vi "Micro-PL v10.2.2.vi"() -> ()   [LabVIEW 2010]
uses:
  drivers/Oxford ITC/ITCAPPS.LLB/ITCSetup.ctl
  drivers/Oxford ITC/ITCSUBS.LLB/ITCIO.ctl
  drivers/Oxford ITC/BUSGEN.LLB/OxfordAddress.ctl
  drivers/Oxford ITC/ITCSUBS.LLB/ITCVersion.ctl
  subvi/ESA-C/TypeDefs/ESA-C Live Controls.ctl
  subvi/ESA-C/TypeDefs/ESA-C Current Values.ctl
  subvi/ESA-C/TypeDefs/ESA-C Connection Settings.ctl
  subvi/ESA-C/TypeDefs/ESA-C Set Positions.ctl
  subvi/ITC503/TypeDefs/ITC503 Settings.ctl
  subvi/ITC503/TypeDefs/ITC503 Current Values.ctl
  subvi/iHR550/TypeDefs/iHR Current Values.ctl
  subvi/iHR550/TypeDefs/iHR Settings.ctl
  subvi/Mapping/TypeDefs/Mapping Spectra Params.ctl
  <vilib>/Utility/miscctls.llb/LVBoundsTypeDef.ctl
  <vilib>/Utility/miscctls.llb/LVPointTypeDef.ctl
  drivers/Horiba Spectrum One 3000V/Lib/CCD_command.llb/Comm Params.ctl
panel:
  out "Copy Drive Target":bool
  in  "CCD3500 Shutter":bool caption="Shutter:"
  out "ITC503 Temp Storage":dbl
  out "Runtime":u32
  out "ITC Gradient Time":i64
  out "Read ITC":bool
  out "Read CCD3500":bool
  out "Read iHR550":bool
  out "Read Drive":bool
  out "Spectrum Properties":cluster{"Position":T1, "Plot Area Size":T1}={"Position"={"Width"=36, "Height"=367}, "Plot Area Size"={"Width"=496, "Height"=264}}
  in  "Auto Folder":path caption="Ausgewählter Pfad"
  out "Int. Time Temp":dbl
  out "Wavelengths (nm)":dbl[](array[numeric])
  out "Measurement Running":bool
  out "ITC503s Running":bool
  out "Drive Running":bool
  out "CCD3500V Running":bool
  out "iHR550 Running":bool
  in  "Exit":bool
  out "iHR550 Status":bool
  out "Drive Status":bool
  out "CCD3500V Status":bool
  out "ITC503 Status":bool
  in  "CCD3500V Connection":T2={"Comm Interface"=1, "BUS"=0, "Address"=5, "Com Port"=0}
  out "Video Running":bool
  out "iHR550 RefNum":refnum<k7> caption="Mono RefNum out"
  out "ITC Setup":T3={"Description"="", "IO Info"={"Address"={"Com Port"=1, "ISOBUS Address"=1, "GPIB Address"=24, "Communication"=enum."ISOBUS"}, "Version"=enum."ITC503", "Ch 1 dec places"=1, "Ch 2 dec places"=1, "Ch 3 dec places"=1, "Ch1 Name"="", "Ch2 Name"="", "Ch3 Name"=""}}
  in  "Register":enum32{"Devices", "Acquisition / Mapping"}(tab)
  out "CCD3500 Temperature":dbl caption="Temp. (°C)" min=10.0 max=160.0 step=0.1 format="%.1f"
  in  "CCD3500V GPIB-Port":i32=5 caption="GPIB-Port" min=1 max=20 step=1 format="%#.0f"
  in  "CCD3500V Connect":bool
  out "CCD Timing":u32 caption="CCD"
  out "ITC Timing":u32 caption="ITC"
  out "Drive Timing":u32 caption="Drive"
  out "iHR550 Timing":u32 caption="iHR550"
  in  "iHR550 Force Init":bool=TRUE
  in  "iHR550 Connect":bool
  in  "iHR550 ID":string(combo)="iHR550" caption="Monochromator ID"
  out "ITC503 Current Values":T7 {"ITC503 Gradient" format="%.2f"; "ITC503 Setpoint" min=-273.0 max=300000.0 step=0.0001 format="%.1f"; "ITC503 I" format="%_1f"; "ITC503 P" format="%_1f"; "ITC503 Temperature" min=0.0 max=1645.0 step=1e-05 format="%.2f"; "ITC503 Heater" min=0.0 max=100.0 step=0.01 scale=0.0..100.0}
  in  "ITC503 Settings":T8={"ITC503 Set Setpoint"=0.0, "ITC503 Set Auto Heater"=TRUE, "ITC503 Set Auto PID"=TRUE, "P"=0.0, "I"=0.0, "D"=0.0} {"D" min=0.0 max=100.0 step=0.1 format="%.1f"; "I" min=0.0 max=100.0 step=0.1 format="%.1f"; "P" min=0.0 max=100.0 step=0.1 format="%.1f"; "ITC503 Set Setpoint" min=-273.0 max=300000.0 step=0.1 format="%.1f"}
  in  "ITC503 Configure":bool
  in  "ITC503 Connect":bool
  in  "ITC503 Selector":u16(ring) caption="Select Device" items=["ITC503s"]
  out "Drive Current Values":T9 {"Position"."Drive Z Position" min=-273.0 max=300000.0 step=0.0001 format="%.1f"; "Position"."Drive Y Position" min=-273.0 max=300000.0 step=0.0001 format="%.1f"; "Position"."Drive X Position" min=-273.0 max=300000.0 step=0.0001 format="%.1f"; "Voltages"."Drive Z Voltage" min=-273.0 max=300000.0 step=0.0001 format="%.1f"; "Voltages"."Drive Y Voltage" min=-273.0 max=300000.0 step=0.0001 format="%.1f"; "Voltages"."Drive X Voltage" min=-273.0 max=300000.0 step=0.0001 format="%.1f"}
  in  "Drive Connection":T10={"Objective GPIB-Port"=4, "Stage GPIB-Port"=4, "Drive Selector"=0, "Drive Velocity (V/s)"=5.0} {"Drive Velocity (V/s)" min=10.0 max=160.0 step=0.1 format="%.1f"; "Drive Selector" items=["Obj.", "Stage"]; "Stage GPIB-Port" min=1 max=20 step=1 format="%#.0f"; "Objective GPIB-Port" min=1 max=20 step=1 format="%#.0f"}
  in  "Drive Connect":bool
  in  "CCD3000 Current Rep.":string="0/0"
  in  "Spectrum Maximize":bool
  out "Spectrum":cluster{dbl[], dbl[]}[](graph)
  in  "Spectrum Load":bool
  in  "Spectrum Save":bool
  in  "Video Show":bool
  in  "Drive GoTo":bool caption="Objective Move Abs."
  in  "Drive New Positions":T11 {"Drive X Set" min=10.0 max=160.0 step=0.1 format="%.1f"; "Drive Z Set" min=10.0 max=160.0 step=0.1 format="%.1f"; "Drive Y Set" min=10.0 max=160.0 step=0.1 format="%.1f"}
  in  "Spectrum Autosave":bool caption="iHR550 Force Init"
  in  "CCD3500 Preview":bool
  in  "CCD3500 Acquire":bool
  in  "Spectra Settings":T12={"Integration Time"=1.0, "Repetitions"=1, "Mapping Spectra"=TRUE} caption="Mapping Spectra Settings" {"Repetitions" min=1 max=100 step=1; "Integration Time" min=0.1 max=6000.0 step=0.1 format="%.1f"}
  in  "Mapping Start":bool
  in  "iHR550 Configure":bool
  in  "iHR Settings":T13={"iHR550 Set Exit Mirror"=2, "iHR550 Set Side Exit"=0.0, "iHR550 Set Front Entrance"=0.0, "iHR550 Set Wavelength"=897.9988, "iHR550 Set Grating"=0, "iHR550 Set Grating Switch"=FALSE, "iHR550 Set Wavelength Switch"=FALSE, "iHR550 Set Mirror Switch"=FALSE, "iHR550 Set Slits Switch"=FALSE} {"iHR550 Set Grating" items=["1800"=1, "600"=2, "150"=3]; "iHR550 Set Wavelength" min=0.0 max=1500.0 step=1.0; "iHR550 Set Side Exit" min=0.0 max=2000.0 step=1.0; "iHR550 Set Exit Mirror" items=["Front"=2, "Side"=3]}
  out "iHR Current Values":T14={"iHR 550 Front Entrance"=0.0, "iHR550 Side Exit"=0.0, "iHR550 Wavelength"=897.9988, "iHR550 Exit Mirror"=2, "iHR550 Grating"="1", "Grating Index"=1} {"iHR550 Exit Mirror" items=["EntranceMirror", "ExitMirror", "Front", "Side"]}
  out "Drive Live Current Values":T9 {"Position"."Drive Z Position" min=-273.0 max=300000.0 step=0.0001 format="%.1f"; "Position"."Drive Y Position" min=-273.0 max=300000.0 step=0.0001 format="%.1f"; "Position"."Drive X Position" min=-273.0 max=300000.0 step=0.0001 format="%.1f"; "Voltages"."Drive Z Voltage" min=-273.0 max=300000.0 step=0.0001 format="%.1f"; "Voltages"."Drive Y Voltage" min=-273.0 max=300000.0 step=0.0001 format="%.1f"; "Voltages"."Drive X Voltage" min=-273.0 max=300000.0 step=0.0001 format="%.1f"}
  in  "Drive Live Controls":T15={"Snapshot"=FALSE, "Move Step"=1.0, "Move Home"=FALSE, "Move Down"=FALSE, "Move Up"=FALSE, "Move Left"=FALSE, "Move Right"=FALSE, "Move Out"=FALSE, "Move In"=FALSE} {"Move Step" min=0.0 max=30.0 step=0.1 format="%.1f"}
  # "Correlation Setup"
  # "Active"
  # "Active"
  # "ITC"
  # "iHR"
  # "Drive"
  # "CCD"
  # "Status"
  # "CCD"
  # "ITC"
  # "iHR"
  # "Drive"
  # "CCD"
  # "Timing"
  # "Monochromator"
  # "Cryostat"
  # "Drives"
  # "Drive Control"
  # "Spectrum"
  # "CCD"
  # "Mapping"
  # "Launch the Spectral Mapping VI and Raman Tool Set 2.0 in a new window."
  # "Monochromator"
  # "XY"
  # "Z"
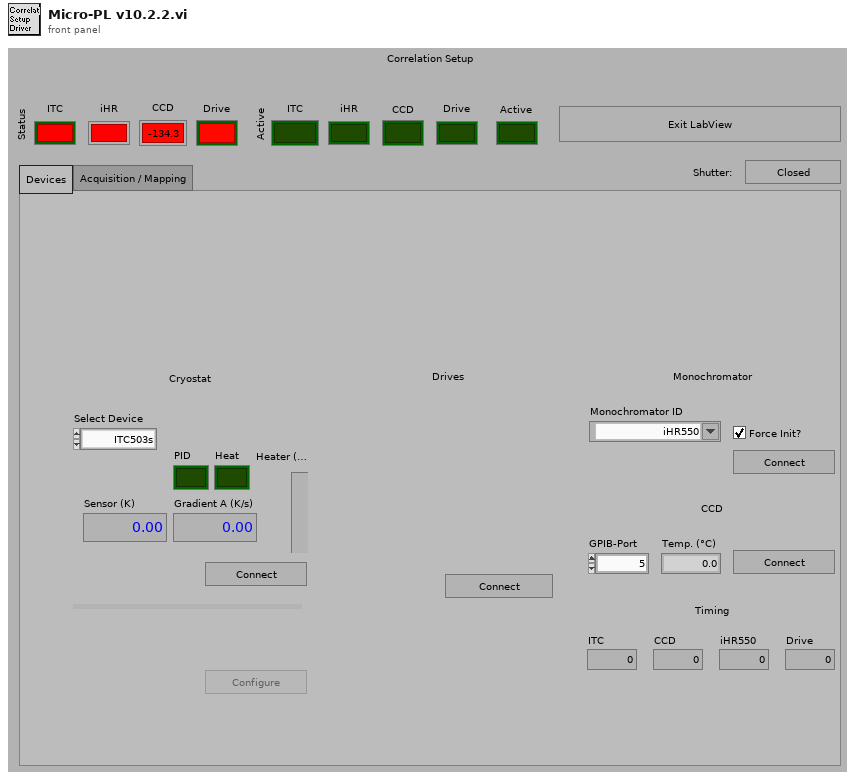
[diagram p1: front panel]
types:
  T1 = typedef "LVBoundsTypeDef.ctl" = cluster{"Width":u32, "Height":u32}
  T2 = cluster{"Comm Interface":u16, "BUS":i16, "Address":i16, "Com Port":i32}
  T3 = typedef "ITCSetup.ctl" = cluster{"Description":string, "IO Info":T4}
  T4 = typedef "ITCIO.ctl" = cluster{"Address":T5, "Version":T6, "Ch 1 dec places":i16, "Ch 2 dec places":i16, "Ch 3 dec places":i16, "Ch1 Name":string, "Ch2 Name":string, "Ch3 Name":string}
  T5 = typedef "OxfordAddress.ctl" = cluster{"Com Port":i32, "ISOBUS Address":i32, "GPIB Address":i16, "Communication":enum16{"RS232", "ISOBUS", "GPIB", "Gateway"}}
  T6 = typedef "ITCVersion.ctl" = enum16{"ITC502", "ITC503", "ITC601"}
  T7 = typedef "ITC503 Current Values.ctl" = cluster{"ITC503 Heater":dbl, "ITC503 Temperature":dbl, "ITC503 P":dbl, "ITC503 I":dbl, "ITC503 D":dbl, "ITC503 Setpoint":dbl, "ITC503 Gradient":dbl, "ITC503 Heater Auto":bool, "ITC503 PID Auto":bool}
  T8 = typedef "ITC503 Settings.ctl" = cluster{"ITC503 Set Setpoint":dbl, "ITC503 Set Auto Heater":bool, "ITC503 Set Auto PID":bool, "P":dbl, "I":dbl, "D":dbl}
  T9 = typedef "ESA-C Current Values.ctl" = cluster{"Voltages":cluster{"Drive X Voltage":dbl, "Drive Y Voltage":dbl, "Drive Z Voltage":dbl}, "Position":cluster{"Drive X Position":dbl, "Drive Y Position":dbl, "Drive Z Position":dbl}}
  T10 = typedef "ESA-C Connection Settings.ctl" = cluster{"Objective GPIB-Port":i32, "Stage GPIB-Port":i32, "Drive Selector":u16, "Drive Velocity (V/s)":dbl}
  T11 = typedef "ESA-C Set Positions.ctl" = cluster{"Drive X Set":dbl, "Drive Y Set":dbl, "Drive Z Set":dbl}
  T12 = typedef "Mapping Spectra Params.ctl" = cluster{"Integration Time":dbl, "Repetitions":u16, "Mapping Spectra":bool}
  T13 = typedef "iHR Settings.ctl" = cluster{"iHR550 Set Exit Mirror":u16, "iHR550 Set Side Exit":dbl, "iHR550 Set Front Entrance":dbl, "iHR550 Set Wavelength":dbl, "iHR550 Set Grating":u16, "iHR550 Set Grating Switch":bool, "iHR550 Set Wavelength Switch":bool, "iHR550 Set Mirror Switch":bool, "iHR550 Set Slits Switch":bool}
  T14 = typedef "iHR Current Values.ctl" = cluster{"iHR 550 Front Entrance":dbl, "iHR550 Side Exit":dbl, "iHR550 Wavelength":dbl, "iHR550 Exit Mirror":i32, "iHR550 Grating":string, "Grating Index":i32}
  T15 = typedef "ESA-C Live Controls.ctl" = cluster{"Snapshot":bool, "Move Step":dbl, "Move Home":bool, "Move Down":bool, "Move Up":bool, "Move Left":bool, "Move Right":bool, "Move Out":bool, "Move In":bool}
  T16 = typedef "LVPointTypeDef.ctl" = cluster{"Horizontal":i16, "Vertical":i16}
  T17 = enum8{"Enabled", "Disabled", "Disabled and Grayed Out"}
  T18 = typedef "Comm Params.ctl" = cluster{"Comm Interface":u16, "BUS":i16, "Address":i16, "Com Port":i32}
  T19 = enum16{"CCD Temperature Z345", "CCD Temperature Z308", "CCD Gain"}
  T20 = cluster{"CCD3000 Connection":T18, "Drive Connection Settings":T10, "ITC503 Current Values":T7, "Wavelengths (nm)":dbl[], "Drive Current Values":T9, "iHR Current Values":T14, "Spectra Settings":T12, "CCD3500 Temperature":dbl, "Simulate Drive 2":bool, "Simulate Spectra 2":bool}
  T21 = cluster{"Drive X Position":dbl, "Drive Y Position":dbl, "Drive Z Position":dbl}
  T22 = cluster{"Intensities":dbl[], "Wavelengths":dbl[]}[]
  T23 = typedef "LVPositionTypeDef.ctl" = cluster{"Left":i32, "Top":i32}
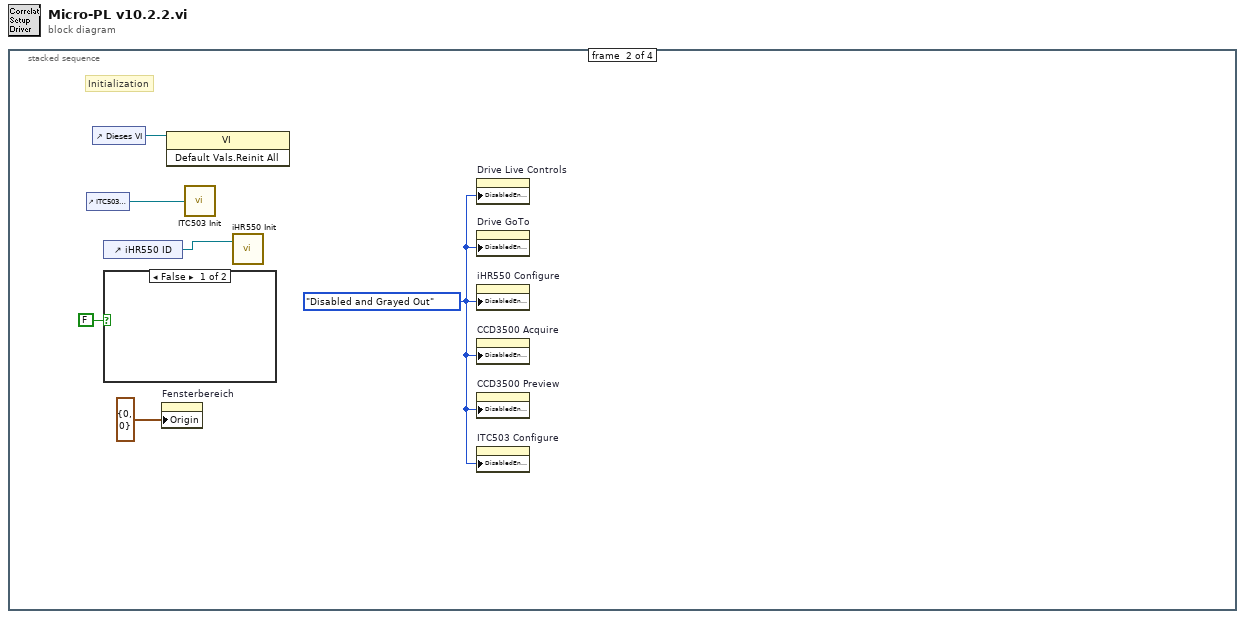
[diagram p0: block diagram]
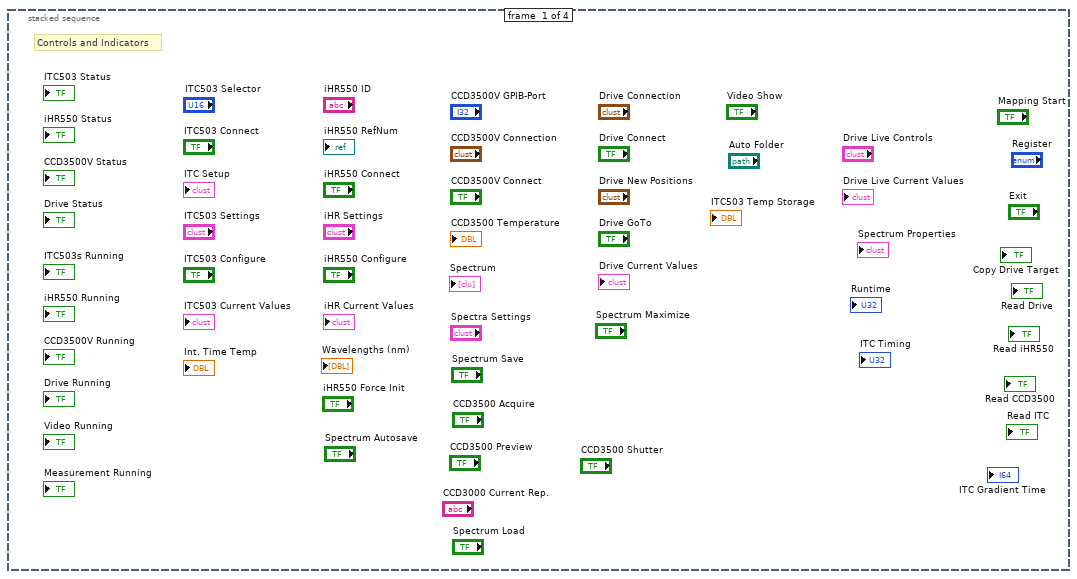
[diagram p2: hidden frame]
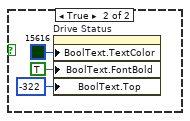
[diagram p3: hidden frame]
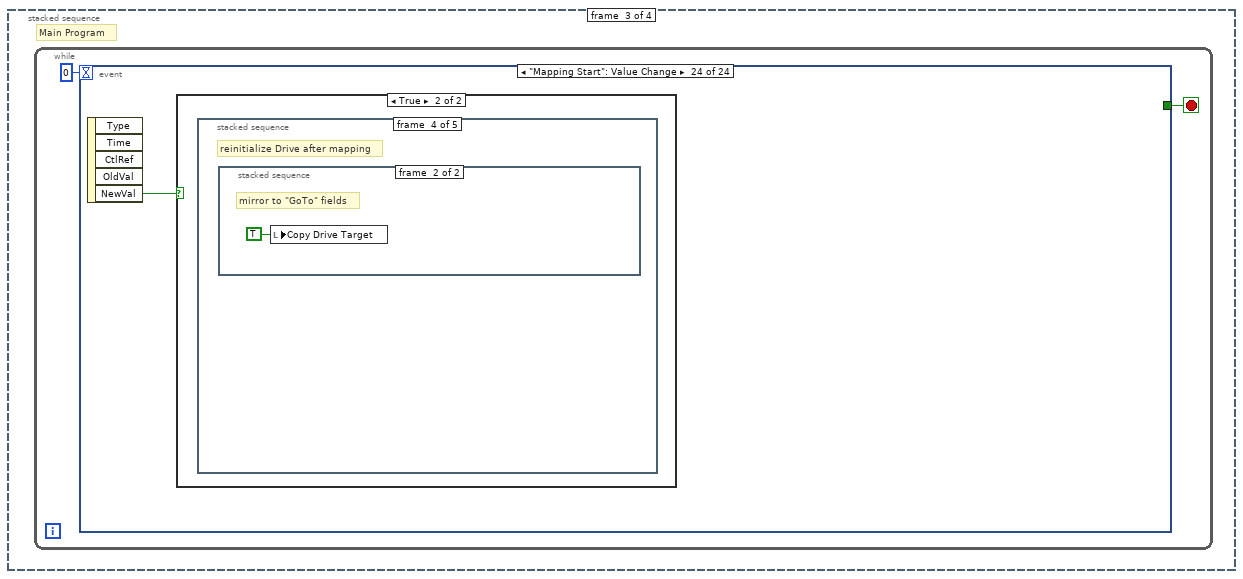
[diagram p4: hidden frame]
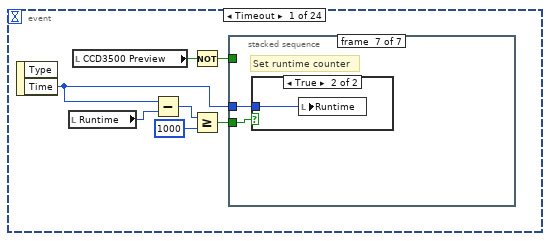
[diagram p5: hidden frame]
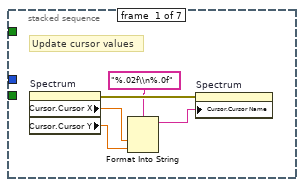
[diagram p6: hidden frame]
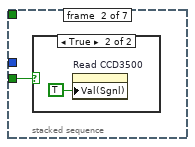
[diagram p7: hidden frame]
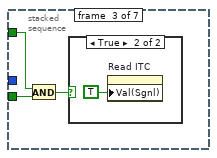
[diagram p9: hidden frame]
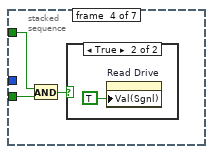
[diagram p11: hidden frame]
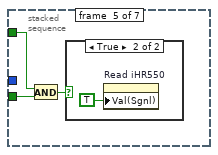
[diagram p13: hidden frame]
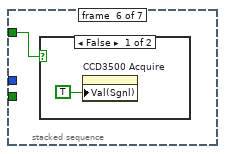
[diagram p15: hidden frame]
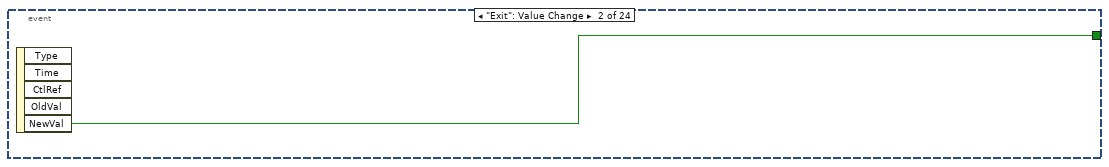
[diagram p18: hidden frame]
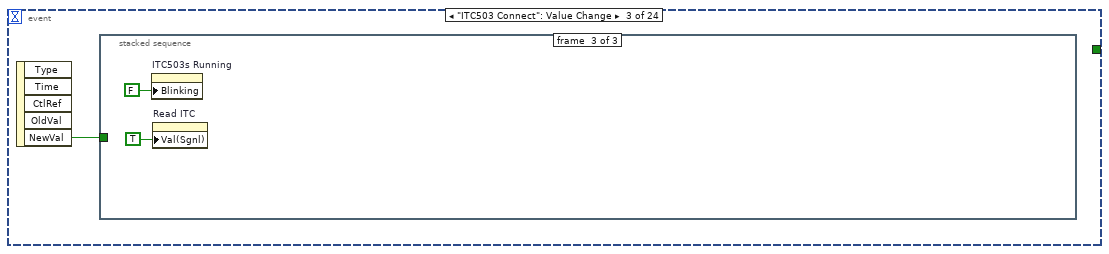
[diagram p19: hidden frame]
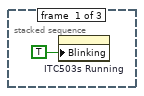
[diagram p20: hidden frame]
diagram:
  n1 = stacked-sequence {
    frame #0 {
      # "Controls and Indicators"
    }
    frame #1 {
      w1 = T17."Disabled and Grayed Out" ("Deaktiviert")
      # "Initialization"
      n2 = control-ref of="ITC503 Selector"() -> (w6:refnum<vi>)
      n3 = control-ref of="Dieses VI"() -> (w5:refnum<vi>)
      n4 = control-ref of="iHR550 ID"() -> (w4:refnum<vi>)
      n5 = case shown="False" FALSE {
        frame False {
        }
        frame True {
          n6 = property on="Drive Status" class="Bool (strict)"("BoolText.TextColor"=u32 15616, "BoolText.FontBold"=TRUE ("Boolescher Text.Schriftart:Fett"), "BoolText.Top"=-322 ("Boolescher Text.Position:Oben")) -> ()  [unwired: 2 in, 2 out]
        }
      }
      n7 = property on="Fensterbereich" class="Pane"("Origin"=T16 {"Horizontal"=0, "Vertical"=0}) -> ()  [unwired: 2 in, 2 out]
      n8 = invoke class="VI" method="Default Vals.Reinit All"(reference=w5) -> ()  [unwired: 2 in, 3 out]
      n9 = call "ITC503 Init.vi"("ITC Selector"=w6) -> ()  [unwired: 1 in]
      n10 = call "iHR550 Init.vi"("Mono ID"=w4) -> ()  [unwired: 2 in]
      n11 = property on="Drive Live Controls" class="Clust (strict)"("DisabledEnum"=w1) -> ()  [unwired: 2 in, 2 out]
      n12 = property on="Drive GoTo" class="Bool (strict)"("DisabledEnum"=w1) -> ()  [unwired: 2 in, 2 out]
      n13 = property on="iHR550 Configure" class="Bool (strict)"("DisabledEnum"=w1) -> ()  [unwired: 2 in, 2 out]
      n14 = property on="CCD3500 Acquire" class="Bool (strict)"("DisabledEnum"=w1) -> ()  [unwired: 2 in, 2 out]
      n15 = property on="CCD3500 Preview" class="Bool (strict)"("DisabledEnum"=w1) -> ()  [unwired: 2 in, 2 out]
      n16 = property on="ITC503 Configure" class="Bool (strict)"("DisabledEnum"=w1) -> ()  [unwired: 2 in, 2 out]
    }
    frame #2 {
      # "Main Program"
      n17 = while "Main-Program" {
        stop <- w11 stop-if-true
        n18 = event shown="[23] \"Mapping Start\": Value Change" {
          selector: _ -> [_ _ _ _ _ _ _ _ _ _ _ _ _ _ _ _ _ _ _ _ _ _ _ _]
          dyn-events: _ -> [_ _ _ _ _ _ _ _ _ _ _ _ _ _ _ _ _ _ _ _ _ _ _ _]
          timeout: 0 -> [_ _ _ _ _ _ _ _ _ _ _ _ _ _ _ _ _ _ _ _ _ _ _ _]
          tunnel: [_ w43 _ _ _ _ _ _ _ _ _ _ _ _ _ _ _ _ _ _ _ _ _ _] -> w11
          event Timeout {
            n19 = event-data() -> ("Time"=w13:u32)  [unwired: 1 in, 1 out]
            n20 = local read "Runtime"() -> (w12:u32)
            n21 = local read "CCD3500 Preview"() -> (w15:bool)
            n22 = Subtract(x=w13, y=w12) -> (x-y=w16:u32)
            n23 = Not(x=w15) -> (.not. x?=w14:bool)
            n24 = Greater Or Equal?(x=w16, y=u32 1000) -> (x >= y?=w17:bool)
            n25 = stacked-sequence {
              tunnel: w17 -> [_ w24 w28 w32 w36 _ w40]
              tunnel: w13 -> [_ _ _ _ _ _ w41]
              tunnel: w14 -> [_ _ w27 w31 w35 w38 _]
              frame #0 {
                # "Update cursor values"
                n26 = property on="Spectrum" class="XYGraph (strict)"() -> (error out=w23:errorcluster, "Cursor.Cursor X"=w22:dbl, "Cursor.Cursor Y"=w21:dbl)  [unwired: 2 in, 1 out]
                n27 = Format Into String(format string="%.02f\\n%.0f", w22, w21) -> (resulting string=w19:string)  [unwired: 2 in, 1 out]
                n28 = property on="Spectrum" class="XYGraph (strict)"(error in=w23, "Cursor.Cursor Name"=w19) -> ()  [unwired: 1 in, 2 out]
              }
              frame #1 {
                n29 = case shown="True" w24 {
                  frame False {
                  }
                  frame True {
                    n30 = property on="Read CCD3500" class="Bool (strict)"("Val(Sgnl)"=TRUE ("Value (Signaling)")) -> ()  [unwired: 2 in, 2 out]
                  }
                }
              }
              frame #2 {
                n31 = And(x=w27, y=w28) -> (x .and. y?=w26:bool)
                n32 = case shown="True" w26 {
                  frame False {
                  }
                  frame True {
                    n33 = property on="Read ITC" class="Bool (strict)"("Val(Sgnl)"=TRUE ("Value (Signaling)")) -> ()  [unwired: 2 in, 2 out]
                  }
                }
              }
              frame #3 {
                n34 = And(x=w31, y=w32) -> (x .and. y?=w30:bool)
                n35 = case shown="True" w30 {
                  frame False {
                  }
                  frame True {
                    n36 = property on="Read Drive" class="Bool (strict)"("Val(Sgnl)"=TRUE ("Value (Signaling)")) -> ()  [unwired: 2 in, 2 out]
                  }
                }
              }
              frame #4 {
                n37 = And(x=w35, y=w36) -> (x .and. y?=w34:bool)
                n38 = case shown="True" w34 {
                  frame False {
                  }
                  frame True {
                    n39 = property on="Read iHR550" class="Bool (strict)"("Val(Sgnl)"=TRUE ("Value (Signaling)")) -> ()  [unwired: 2 in, 2 out]
                  }
                }
              }
              frame #5 {
                n40 = case shown="False" w38 {
                  frame False {
                    n41 = property on="CCD3500 Acquire" class="Bool (strict)"("Val(Sgnl)"=TRUE ("Wert (signalisierend)")) -> ()  [unwired: 2 in, 2 out]
                  }
                  frame True {
                  }
                }
              }
              frame #6 {
                # "Set runtime counter"
                n42 = case shown="True" w40 {
                  tunnel: w41 -> [_ w42]
                  frame False {
                  }
                  frame True {
                    n43 = local write "Runtime"(w42) -> ()
                  }
                }
              }
            }
          }
          event "Exit": Value Change {
            n44 = event-data() -> ("NewVal"=w43:bool)  [unwired: 1 in, 4 out]
          }
          event "ITC503 Connect": Value Change {
            n45 = event-data() -> ("NewVal"=w44:bool)  [unwired: 1 in, 4 out]
            n46 = stacked-sequence {
              tunnel: w44 -> [_ w46 _]
              frame #0 {
                n47 = property on="ITC503s Running" class="Bool (strict)"("Blinking"=TRUE ("Blinkend")) -> ()  [unwired: 2 in, 2 out]
              }
              frame #1 {
                n48 = case shown="True" w46 {
                  selector: w46 -> [w51 _]
                  tunnel: [w51 w58] -> w48
                  frame False {
                    # "disconnect"
                    n49 = control-ref of="ITC503s Running"() -> (w52:refnum<vi>)
                    n50 = property class="Bool (strict)"(reference=w52, "Blinking"=w51, "Value"=w51) -> ()  [unwired: 1 in, 2 out]
                  }
                  frame True {
                    # "connect"
                    n51 = local read "ITC503 Selector"() -> (w59:u16)
                    n52 = call "ITC503 Connect.vi"("ITC Selector"=w59) -> ("ITC Setup"=w57:T3, "Connected"=w58:bool)
                    n53 = local write "ITC Setup"(w57) -> ()
                    n54 = call "ITC503 Get Values.vi"("ITC Setup"=w57) -> ("ITC503 Current Values"=w56:T7)  [unwired: 1 in, 1 out]
                    n55 = Unbundle By Name(w56) -> ("ITC503 Setpoint"=w53:dbl)
                    n56 = Bundle By Name(cluster=T8 {"ITC503 Set Setpoint"=0.0, "ITC503 Set Auto Heater"=TRUE, "ITC503 Set Auto PID"=TRUE, "P"=0.0, "I"=0.0, "D"=0.0} ("ITC503 Settings"), "ITC503 Set Setpoint"=w53) -> (w54:T8)
                    n57 = local write "ITC503 Settings"(w54) -> ()
                  }
                }
                n58 = case shown="False" w48 {
                  tunnel: [T17."Disabled and Grayed Out" ("Deaktiviert") T17."Enabled" ("Deaktiviert")] -> w47
                  frame False {
                  }
                  frame True {
                  }
                }
                n59 = local write "ITC503 Status"(w48) -> ()
                n60 = local write "ITC503 Connect"(w48) -> ()
                n61 = property on="ITC503 Configure" class="Bool (strict)"("DisabledEnum"=w47) -> ()  [unwired: 2 in, 2 out]
              }
              frame #2 {
                n62 = property on="ITC503s Running" class="Bool (strict)"("Blinking"=FALSE ("Blinkend")) -> ()  [unwired: 2 in, 2 out]
                n63 = property on="Read ITC" class="Bool (strict)"("Val(Sgnl)"=TRUE ("Wert (signalisierend)")) -> ()  [unwired: 2 in, 2 out]
              }
            }
          }
          event "Read ITC": Value Change {
            n64 = event-data() -> ("Time"=w63:u32, "NewVal"=w67:bool)  [unwired: 1 in, 3 out]
            n65 = local read "ITC503 Status"() -> (w66:bool)
            n66 = control-ref of="ITC503s Running"() -> (w64:refnum<vi>)
            n67 = And(x=w66, y=w67) -> (x .and. y?=w65:bool)
            n68 = case shown="True" w65 {
              tunnel: w64 -> [w69 w73]
              tunnel: w63 -> [_ w72]
              tunnel: [u32 0 w71] -> w62
              frame False {
                n69 = property class="Bool (strict)"(reference=w69, "BoolText.Text"="" ("Boolescher Text.Text")) -> ()  [unwired: 1 in, 2 out]
              }
              frame True {
                n70 = stacked-sequence {
                  seq-local: [_ w78 _ _] -> [_ _ w95 _]
                  seq-local: [w74 _ _ _] -> [_ _ _ w101]
                  tunnel: w73 -> [_ _ w88 _]
                  tunnel: w72 -> [_ w79 _ _]
                  tunnel: [_ _ _ w102] -> w71
                  frame #0 {
                    n71 = Tick Count (ms)() -> (millisecond timer value=w74:u32)
                  }
                  frame #1 {
                    n72 = local read "ITC Setup"() -> (w86:T3)
                    n73 = local read "ITC Gradient Time"() -> (w83:i64)
                    n74 = call "ITC503 Get Values.vi"("ITC Setup"=w86) -> ("ITC503 Current Values"=w78:T7)  [unwired: 1 in, 1 out]
                    n75 = local read "ITC503 Temp Storage"() -> (w77:dbl)
                    n76 = Unbundle By Name(w78) -> ("ITC503 Temperature"=w75:dbl)
                    n77 = Subtract(x=w79, y=w83) -> (x-y=w82:i64)
                    n78 = Divide(x=w82, y=i64 1000) -> (x/y=w80:dbl)
                    n79 = Subtract(x=w75, y=w77) -> (x-y=w76:dbl)
                    n80 = Divide(x=w76, y=w80) -> (x/y=w85:dbl)
                    n81 = Bundle By Name(cluster=w78, "ITC503 Gradient"=w85) -> (w84:T7)
                    n82 = local write "ITC503 Current Values"(w84) -> ()
                  }
                  frame #2 {
                    n83 = Unbundle By Name(w95) -> ("ITC503 Temperature"=w87:dbl, "ITC503 Setpoint"=w96:dbl)
                    n84 = Subtract(x=w87, y=w96) -> (x-y=w97:dbl)
                    n85 = Number To Fractional String(number=w87, precision (6)=i16 2 ("Genauigkeit (6)")) -> (F-format string=w91:string)  [unwired: 2 in]
                    n86 = Absolute Value(x=w97) -> (abs(x)=w98:dbl)
                    n87 = String Subset(string=w91, length (rest)=5 ("Länge (Rest)")) -> (substring=w89:string)  [unwired: 1 in]
                    n88 = Greater?(x=w98, y=2.0) -> (0:w94:bool)
                    n89 = Not(x=w94) -> (.not. x?=w93:bool)
                    n90 = property class="Bool (strict)"(reference=w88, "Blinking"=w94, "Value"=w93, "BoolText.Text"=w89) -> ()  [unwired: 1 in, 2 out]
                    n91 = local write "ITC503 Temp Storage"(w87) -> ()
                  }
                  frame #3 {
                    n92 = Tick Count (ms)() -> (millisecond timer value=w100:u32)
                    n93 = local write "ITC Gradient Time"(w100) -> ()
                    n94 = Subtract(x=w100, y=w101) -> (x-y=w102:u32)
                  }
                }
              }
            }
            n95 = local write "ITC Timing"(w62) -> ()
          }
          event "iHR550 Connect": Value Change {
            n96 = event-data() -> ("NewVal"=w103:bool)  [unwired: 1 in, 4 out]
            n97 = stacked-sequence {
              tunnel: w103 -> [_ w106 _]
              frame #0 {
                n98 = property on="iHR550 Running" class="Bool (strict)"("Blinking"=TRUE ("Blinkend")) -> ()  [unwired: 2 in, 2 out]
              }
              frame #1 {
                n99 = case shown="True" w106 {
                  selector: w106 -> [w110 _]
                  tunnel: [w110 w123] -> w105
                  frame False {
                    # "disconnect"
                  }
                  frame True {
                    # "connect"
                    n100 = local read "iHR550 Force Init"() -> (w121:bool)
                    n101 = control-ref of="iHR550 Set Grating"() -> (w122:refnum<vi>)
                    n102 = local read "iHR550 ID"() -> (w124:string)
                    n103 = call "iHR550 Connect.vi"("Force\nInitialization"=w121, "Grating Selector"=w122, "Mono ID"=w124) -> ("Initialized"=w123:bool, "iHR550 RefNum"=w120:refnum<k7>)  [unwired: 2 in, 4 out]
                    n104 = local write "iHR550 RefNum"(w120) -> ()
                    n105 = call "iHR550 Read Values.vi"("JYMONOLib.IJYMonoReqd"=w120) -> ("iHR Current Values"=w112:T14)  [unwired: 1 in]
                    n106 = local write "iHR Current Values"(w112) -> ()
                    n107 = Unbundle By Name(w112) -> ("iHR 550 Front Entrance"=w118:dbl, "iHR550 Side Exit"=w117:dbl, "iHR550 Wavelength"=w116:dbl, "iHR550 Exit Mirror"=w115:i32, "Grating Index"=w113:i32)
                    n108 = call "iHR550 Convert Axis.vi"("iHR Current Values"=w112) -> ("Wavelengths (nm)"=w111:dbl[])
                    n109 = local write "Wavelengths (nm)"(w111) -> ()
                    n110 = Bundle By Name(cluster=T13 {"iHR550 Set Exit Mirror"=0, "iHR550 Set Side Exit"=0.0, "iHR550 Set Front Entrance"=0.0, "iHR550 Set Wavelength"=0.0, "iHR550 Set Grating"=0, "iHR550 Set Grating Switch"=FALSE, "iHR550 Set Wavelength Switch"=FALSE, "iHR550 Set Mirror Switch"=FALSE, "iHR550 Set Slits Switch"=FALSE} ("iHR Settings"), "iHR550 Set Front Entrance"=w118, "iHR550 Set Side Exit"=w117, "iHR550 Set Wavelength"=w116, "iHR550 Set Exit Mirror"=w115, "iHR550 Set Grating"=w113) -> (w114:T13)
                    n111 = local write "iHR Settings"(w114) -> ()
                  }
                }
                n112 = local write "iHR550 Status"(w105) -> ()
                n113 = local write "iHR550 Connect"(w105) -> ()
                n114 = case shown="False" w105 {
                  tunnel: [T17."Disabled and Grayed Out" ("Deaktiviert") T17."Enabled" ("Deaktiviert")] -> w107
                  frame False {
                  }
                  frame True {
                  }
                }
                n115 = property on="iHR550 Configure" class="Bool (strict)"("DisabledEnum"=w107) -> ()  [unwired: 2 in, 2 out]
              }
              frame #2 {
                n116 = local write "iHR550 Force Init"(FALSE ("iHR550 Force Init")) -> ()
                n117 = property on="iHR550 Running" class="Bool (strict)"("Blinking"=FALSE ("Blinkend")) -> ()  [unwired: 2 in, 2 out]
                n118 = property on="Read iHR550" class="Bool (strict)"("Val(Sgnl)"=TRUE ("Wert (signalisierend)")) -> ()  [unwired: 2 in, 2 out]
              }
            }
          }
          event "Read iHR550": Value Change {
            n119 = event-data() -> ("NewVal"=w131:bool)  [unwired: 1 in, 4 out]
            n120 = local read "iHR550 Status"() -> (w130:bool)
            n121 = And(x=w130, y=w131) -> (x .and. y?=w129:bool)
            n122 = case shown="False" w129 {
              tunnel: [u32 0 w133] -> w128
              frame False {
              }
              frame True {
                n123 = stacked-sequence {
                  seq-local: [w134 _ _] -> [_ _ w137]
                  tunnel: [_ _ w138] -> w133
                  frame #0 {
                    n124 = Tick Count (ms)() -> (millisecond timer value=w134:u32)
                  }
                  frame #1 {
                    n125 = local read "iHR550 RefNum"() -> (w136:refnum<k7>)
                    n126 = call "iHR550 Read Values.vi"("JYMONOLib.IJYMonoReqd"=w136) -> ("iHR Current Values"=w135:T14)  [unwired: 1 in]
                    n127 = local write "iHR Current Values"(w135) -> ()
                  }
                  frame #2 {
                    n128 = Tick Count (ms)() -> (millisecond timer value=w139:u32)
                    n129 = Subtract(x=w139, y=w137) -> (x-y=w138:u32)
                  }
                }
              }
            }
            "iHR550 Timing" <- w128
          }
          event "CCD3500V Connect": Value Change {
            n130 = event-data() -> ("NewVal"=w140:bool)  [unwired: 1 in, 4 out]
            n131 = stacked-sequence {
              tunnel: w140 -> [_ w142 _]
              frame #0 {
                n132 = property on="CCD3500V Running" class="Bool (strict)"("Blinking"=TRUE ("Blinkend")) -> ()  [unwired: 2 in, 2 out]
              }
              frame #1 {
                n133 = case shown="True" w142 {
                  selector: w142 -> [w148 _]
                  tunnel: [w148 w149] -> w144
                  frame False {
                    # "disconnect"
                    n134 = local read "CCD3500V Connection"() -> (w147:T2)
                    n135 = call "CCDSTOP.VI"("Comm Params"=w147) -> ()  [unwired: 1 out]
                  }
                  frame True {
                    # "connect"
                    n136 = stacked-sequence {
                      seq-local: [_ w153 _] -> [_ _ w155]
                      tunnel: [_ w154 _] -> w149
                      frame #0 {
                        n137 = local read "CCD3500V GPIB-Port"() -> (w151:i32)
                        n138 = Bundle By Name(cluster=T18 {"Comm Interface"=1, "BUS"=0, "Address"=5, "Com Port"=1} ("Comm Params"), "Address"=w151) -> (w152:T18)
                        n139 = local write "CCD3500V Connection"(w152) -> ()
                      }
                      frame #1 {
                        n140 = local read "CCD3500V Connection"() -> (w153:T2)
                        n141 = call "CCD3000 Initialize.vi"("Comm Params"=w153) -> ("Success"=w154:bool)  [unwired: 9 in, 1 out]
                      }
                      frame #2 {
                        n142 = local read "Spectra Settings"() -> (w156:T12)
                        n143 = Unbundle By Name(w156) -> ("Integration Time"=w157:dbl)
                        n144 = local write "Int. Time Temp"(w157) -> ()
                        n145 = call "CCD3000 Prepare Acquisition.vi"("Mapping Spectra Settings"=w156, "Comm Params"=w155) -> ()  [unwired: 4 in]
                      }
                    }
                  }
                }
                n146 = local write "CCD3500V Connect"(w144) -> ()
                n147 = local write "CCD3500V Status"(w144) -> ()
                n148 = case shown="False" w144 {
                  tunnel: [T17."Disabled and Grayed Out" ("Deaktiviert") T17."Enabled" ("Deaktiviert")] -> w143
                  frame False {
                  }
                  frame True {
                  }
                }
                n149 = property on="CCD3500V Status" class="Bool (strict)"("BoolText.Visible"=w144) -> ()  [unwired: 2 in, 2 out]
                n150 = property on="CCD3500 Acquire" class="Bool (strict)"("DisabledEnum"=w143) -> ()  [unwired: 2 in, 2 out]
                n151 = property on="CCD3500 Preview" class="Bool (strict)"("DisabledEnum"=w143) -> ()  [unwired: 2 in, 2 out]
              }
              frame #2 {
                n152 = property on="Read CCD3500" class="Bool (strict)"("Val(Sgnl)"=TRUE ("Wert (signalisierend)")) -> ()  [unwired: 2 in, 2 out]
                n153 = property on="CCD3500V Running" class="Bool (strict)"("Blinking"=FALSE ("Blinkend")) -> ()  [unwired: 2 in, 2 out]
              }
            }
          }
          event "Read CCD3500": Value Change {
            n154 = event-data() -> ("NewVal"=w163:bool)  [unwired: 1 in, 4 out]
            n155 = local read "CCD3500V Status"() -> (w162:bool)
            n156 = And(x=w162, y=w163) -> (x .and. y?=w161:bool)
            n157 = case shown="False" w161 {
              tunnel: [u32 0 w165] -> w160
              frame False {
              }
              frame True {
                n158 = stacked-sequence {
                  seq-local: [_ w167 _ _] -> [_ _ w176 _]
                  seq-local: [w166 _ _ _] -> [_ _ _ w183]
                  tunnel: [_ _ _ w184] -> w165
                  frame #0 {
                    n159 = Tick Count (ms)() -> (millisecond timer value=w166:u32)
                  }
                  frame #1 {
                    n160 = local read "CCD3500V Connection"() -> (w171:T2)
                    n161 = call "PROPGET.VI"("CCD Prop ID"=T19."CCD Temperature Z345", "Comm Params"=w171) -> ("Output Param"=w169:dbl)  [unwired: 1 out]
                    n162 = Subtract(x=w169, y=273.15) -> (x-y=w167:dbl)
                    n163 = local write "CCD3500 Temperature"(w167) -> ()
                  }
                  frame #2 {
                    n164 = Greater?(x=w176, y=-115.0) -> (0:w172:bool)
                    n165 = case shown="True" w172 {
                      selector: w172 -> [w180 w182]
                      tunnel: [cluster{u32, u32}[] [{16713728, 16713728}, {6618880, 6618880}] ("Farben [4]") cluster{u32, u32}[] [{16713728, 16713728}] ("Farben [4]")] -> w173
                      tunnel: [w180 w182] -> w175
                      frame False {
                      }
                      frame True {
                      }
                    }
                    n166 = Number To Fractional String(number=w176, precision (6)=i16 1 ("Genauigkeit (6)")) -> (F-format string=w174:string)  [unwired: 2 in]
                    n167 = property on="CCD3500V Status" class="Bool (strict)"("Blinking"=w175, "BoolText.Text"=w174, "Colors [4]"=w173) -> ()  [unwired: 2 in, 2 out]
                  }
                  frame #3 {
                    n168 = Tick Count (ms)() -> (millisecond timer value=w185:u32)
                    n169 = Subtract(x=w185, y=w183) -> (x-y=w184:u32)
                  }
                }
              }
            }
            "CCD Timing" <- w160
          }
          event "Drive Connect": Value Change {
            n170 = event-data() -> ("NewVal"=w186:bool)  [unwired: 1 in, 4 out]
            n171 = stacked-sequence {
              tunnel: w186 -> [_ w190 _]
              frame #0 {
                n172 = property on="Drive Running" class="Bool (strict)"("Blinking"=TRUE ("Blinkend")) -> ()  [unwired: 2 in, 2 out]
              }
              frame #1 {
                n173 = local read "Drive Connection"() -> (w191:T10)
                n174 = Not(x=w190) -> (.not. x?=w192:bool)
                n175 = call "ESA-C Connect.vi"("Remote=F /Local=T"=w192, "Drive Connection Settings"=w191) -> ("Success"=w193:bool)  [unwired: 2 in]
                n176 = Exclusive Or(1:w192, 2:w193) -> (0:w194:bool)
                n177 = local write "Drive Connect"(w194) -> ()
                n178 = local write "Drive Status"(w194) -> ()
                n179 = case shown="False" w194 {
                  tunnel: [T17."Disabled and Grayed Out" ("Deaktiviert") T17."Enabled" ("Deaktiviert")] -> w189
                  tunnel: ["" ("Boolescher Text.Text") w197] -> w188
                  frame False {
                  }
                  frame True {
                    n180 = property on="Drive Selector" class="Ring (strict)"() -> ("RingText.Text"=w197:string)  [unwired: 2 in, 2 out]
                  }
                }
                n181 = property on="Drive Live Controls" class="Clust (strict)"("DisabledEnum"=w189) -> ()  [unwired: 2 in, 2 out]
                n182 = property on="Drive Status" class="Bool (strict)"("BoolText.Text"=w188) -> ()  [unwired: 2 in, 2 out]
                n183 = property on="Drive GoTo" class="Bool (strict)"("DisabledEnum"=w189) -> ()  [unwired: 2 in, 2 out]
              }
              frame #2 {
                n184 = property on="Drive Running" class="Bool (strict)"("Blinking"=FALSE ("Blinkend")) -> ()  [unwired: 2 in, 2 out]
                n185 = property on="Read Drive" class="Bool (strict)"("Val(Sgnl)"=TRUE ("Wert (signalisierend)")) -> ()  [unwired: 2 in, 2 out]
              }
            }
          }
          event "Read Drive": Value Change {
            n186 = event-data() -> ("NewVal"=w204:bool)  [unwired: 1 in, 4 out]
            n187 = local read "Drive Status"() -> (w203:bool)
            n188 = And(x=w203, y=w204) -> (x .and. y?=w202:bool)
            n189 = case shown="True" w202 {
              tunnel: [u32 0 w206] -> w201
              frame False {
              }
              frame True {
                n190 = stacked-sequence {
                  seq-local: [w207 _ _ _] -> [_ _ _ w213]
                  tunnel: [_ _ _ w212] -> w206
                  frame #0 {
                    n191 = Tick Count (ms)() -> (millisecond timer value=w207:u32)
                  }
                  frame #1 {
                    n192 = local read "Drive Connection"() -> (w209:T10)
                    n193 = call "ESA-C Get Values.vi"("Drive Connection Settings"=w209) -> ("Drive Current Values"=w208:T9)
                    n194 = local write "Drive Live Current Values"(w208) -> ()
                    n195 = local write "Drive Current Values"(w208) -> ()
                  }
                  frame #2 {
                    n196 = local read "Copy Drive Target"() -> (w210:bool)
                    n197 = case shown="True" w210 {
                      frame False {
                      }
                      frame True {
                        n198 = property on="Copy Drive Target" class="Bool (strict)"("Val(Sgnl)"=TRUE ("Value (Signaling)")) -> ()  [unwired: 2 in, 2 out]
                      }
                    }
                  }
                  frame #3 {
                    n199 = Tick Count (ms)() -> (millisecond timer value=w214:u32)
                    n200 = Subtract(x=w214, y=w213) -> (x-y=w212:u32)
                  }
                }
              }
            }
            "Drive Timing" <- w201
          }
          event "Copy Drive Target": Value Change {
            # "this event is triggered after drive readout\nit should usually not be triggered directly by signaling"
            n201 = event-data() -> ("NewVal"=w215:bool)  [unwired: 1 in, 4 out]
            n202 = case shown="True" w215 {
              frame False {
              }
              frame True {
                n203 = stacked-sequence {
                  frame #0 {
                    n204 = local read "Drive Current Values"() -> (w217:T9)
                    n205 = Unbundle By Name(w217) -> ("Position"=w216:T21)
                    n206 = local write "Drive New Positions"(w216) -> ()
                  }
                  frame #1 {
                    n207 = local write "Copy Drive Target"(FALSE ("Copy Drive Target")) -> ()
                  }
                }
              }
            }
          }
          event "Video Show": Value Change {
            n208 = event-data() -> ("NewVal"=w219:bool)  [unwired: 1 in, 4 out]
            n209 = case shown="False" w219 {
              frame False {
                n210 = call "Video Close.vi"() -> ()  [unwired: 11 in, 1 out]
              }
              frame True {
                n211 = call "Video Open.vi"() -> ()  [unwired: 11 in, 1 out]
              }
            }
          }
          event "ITC503 Configure": Value Change {
            n212 = event-data() -> ("NewVal"=w220:bool)  [unwired: 1 in, 4 out]
            n213 = stacked-sequence {
              tunnel: w220 -> [_ w222 _]
              frame #0 {
                n214 = property on="ITC503s Running" class="Bool (strict)"("Blinking"=TRUE ("Blinkend")) -> ()  [unwired: 2 in, 2 out]
              }
              frame #1 {
                n215 = local read "ITC503 Status"() -> (w224:bool)
                n216 = And(x=w224, y=w222) -> (x .and. y?=w223:bool)
                n217 = case shown="True" w223 {
                  frame False {
                  }
                  frame True {
                    n218 = local read "ITC503 Settings"() -> (w225:T8)
                    n219 = local read "ITC Setup"() -> (w226:T3)
                    n220 = call "ITC503 Set Values.vi"("Set Channel"=i16 1, "ITC503 Settings"=w225, "ITC Setup"=w226) -> ()  [unwired: 2 in]
                  }
                }
              }
              frame #2 {
                w229 = FALSE ("Blinkend")
                n221 = local write "ITC503 Configure"(w229) -> ()
                n222 = property on="ITC503s Running" class="Bool (strict)"("Blinking"=w229) -> ()  [unwired: 2 in, 2 out]
                n223 = property on="Read ITC" class="Bool (strict)"("Val(Sgnl)"=TRUE ("Wert (signalisierend)")) -> ()  [unwired: 2 in, 2 out]
              }
            }
          }
          event "iHR550 Configure": Value Change {
            n224 = event-data() -> ("NewVal"=w230:bool)  [unwired: 1 in, 4 out]
            n225 = stacked-sequence {
              tunnel: w230 -> [_ w232 _]
              frame #0 {
                n226 = property on="iHR550 Running" class="Bool (strict)"("Blinking"=TRUE ("Blinkend")) -> ()  [unwired: 2 in, 2 out]
              }
              frame #1 {
                n227 = local read "iHR550 Status"() -> (w234:bool)
                n228 = local read "iHR550 RefNum"() -> (w235:refnum<k7>)
                n229 = And(x=w234, y=w232) -> (x .and. y?=w233:bool)
                n230 = case shown="True" w233 {
                  tunnel: w235 -> [_ w236]
                  frame False {
                  }
                  frame True {
                    n231 = stacked-sequence {
                      seq-local: [_ w241 _] -> [_ _ w244]
                      tunnel: w236 -> [w237 w242 _]
                      frame #0 {
                        w240 = u16 2 items=["Front"=2, "Side"=3] ("Entrance Mirror")
                        n232 = local read "iHR Settings"() -> (w238:T13)
                        n233 = call "iHR550 Set Values.vi"("Refnum out"=w237, "Entrance Mirror"=w240, "Target\nSide Entrance"=0.0 ("Target\nSide Entrance"), "iHR Settings"=w238) -> ()  [unwired: 11 in, 1 out]
                      }
                      frame #1 {
                        n234 = call "iHR550 Read Values.vi"("JYMONOLib.IJYMonoReqd"=w242) -> ("iHR Current Values"=w241:T14)  [unwired: 1 in]
                        n235 = local write "iHR Current Values"(w241) -> ()
                      }
                      frame #2 {
                        n236 = call "iHR550 Convert Axis.vi"("iHR Current Values"=w244) -> ("Wavelengths (nm)"=w243:dbl[])
                        n237 = local write "Wavelengths (nm)"(w243) -> ()
                      }
                    }
                  }
                }
              }
              frame #2 {
                w246 = FALSE ("Blinkend")
                n238 = property on="Read iHR550" class="Bool (strict)"("Val(Sgnl)"=TRUE ("Wert (signalisierend)")) -> ()  [unwired: 2 in, 2 out]
                n239 = local write "iHR550 Configure"(w246) -> ()
                n240 = property on="iHR550 Running" class="Bool (strict)"("Blinking"=w246) -> ()  [unwired: 2 in, 2 out]
              }
            }
          }
          event "CCD3500 Preview": Value Change {
            n241 = event-data() -> ("NewVal"=w247:bool)  [unwired: 1 in, 4 out]
            n242 = case shown="True" w247 {
              frame False {
              }
              frame True {
                n243 = property on="CCD3500 Acquire" class="Bool (strict)"("Val(Sgnl)"=TRUE ("Wert (signalisierend)")) -> ()  [unwired: 2 in, 2 out]
              }
            }
          }
          event "CCD3500 Acquire": Value Change {
            n244 = event-data() -> ("NewVal"=w249:bool)  [unwired: 1 in, 4 out]
            n245 = stacked-sequence {
              tunnel: w249 -> [w250 _]
              frame #0 {
                n246 = case shown="True" w250 {
                  frame False {
                  }
                  frame True {
                    n247 = local read "CCD3500V Connection"() -> (w251:T2)
                    n248 = local read "Spectra Settings"() -> (w252:T12)
                    n249 = stacked-sequence {
                      tunnel: w252 -> [w255 w267 _]
                      tunnel: w251 -> [w254 w263 _]
                      frame #0 {
                        # "prepare acquisition if settings changed"
                        n250 = Unbundle By Name(w255) -> ("Integration Time"=w253:dbl)
                        n251 = local read "Int. Time Temp"() -> (w256:dbl)
                        n252 = Equal?(x=w253, y=w256) -> (x = y?=w257:bool)
                        n253 = case shown="False" w257 {
                          tunnel: w256 -> [_ _]
                          tunnel: w255 -> [w260 _]
                          tunnel: w254 -> [w259 _]
                          tunnel: w253 -> [w258 _]
                          frame False {
                            n254 = local write "Int. Time Temp"(w258) -> ()
                            n255 = call "CCD3000 Prepare Acquisition.vi"("Mapping Spectra Settings"=w260, "Comm Params"=w259) -> ()  [unwired: 4 in]
                          }
                          frame True {
                          }
                        }
                      }
                      frame #1 {
                        n256 = local read "CCD3500 Preview"() -> (w266:bool)
                        n257 = Unbundle By Name(w267) -> ("Repetitions"=w264:u16)
                        n258 = Select(t=i8 1, s=w266, f=w264) -> (s? t:f=w262:u16)
                        n259 = for {
                          N: w262 -> [w272]
                          tunnel: w263 -> [w284]
                          shift-right: [w279] -> _
                          shift-left: u16[][] [] -> [w282]
                          i -> [w273]
                          stop <- w278 continue-if-true
                          n260 = control-ref of="CCD3500 Acquire"() -> (w277:refnum<vi>)
                          n261 = control-ref of="CCD3500V Running"() -> (w276:refnum<vi>)
                          n262 = call "CCD3000 Spectral Acquisition.vi"("Acquire"=w277, "Running"=w276, "Comm Params"=w284) -> ("Raw-Spectrum"=w283:u16[])  [unwired: 6 in, 2 out]
                          n263 = Number To Decimal String(number=w272) -> (decimal integer string=w271:string)  [unwired: 1 in]
                          n264 = Build Array (concatenate)(w283, w282) -> (w279:u16[][])
                          n265 = Increment(x=w273) -> (x+1=w269:i32)
                          n266 = Number To Decimal String(number=w269) -> (decimal integer string=w270:string)  [unwired: 1 in]
                          n267 = local read "Wavelengths (nm)"() -> (w281:dbl[])
                          n268 = Concatenate Strings(w270, "/" ("string"), w271) -> (w275:string)
                          n269 = call "CCD3000 Average Spectra.vi"("Repetitions"=w269, "Raw Spectra"=w279) -> ("Raw Spectrum"=w280:dbl[])
                          n270 = local read "CCD3500 Acquire"() -> (w278:bool)
                          n271 = local write "CCD3000 Current Rep."(w275) -> ()
                          n272 = call "CCD3000 Pixel to Wavelength v10.1.0.vi"("Wavelengths (nm)"=w281, "Raw Spectrum"=w280) -> ("Spectrum-Cluster"=w268:T22)  [unwired: 1 out]
                          n273 = local write "Spectrum"(w268) -> ()
                        }
                      }
                      frame #2 {
                        n274 = local read "Spectrum Autosave"() -> (w285:bool)
                        n275 = case shown="True" w285 {
                          frame False {
                          }
                          frame True {
                            n276 = property on="Spectrum Save" class="Bool (strict)"("Val(Sgnl)"=TRUE ("Value (Signaling)")) -> ()  [unwired: 2 in, 2 out]
                          }
                        }
                      }
                    }
                  }
                }
              }
              frame #1 {
                n277 = local write "CCD3500 Acquire"(FALSE ("Blinkend")) -> ()
                n278 = local write "CCD3000 Current Rep."("0/0" ("CCD3000 Current Rep.")) -> ()
              }
            }
          }
          event "CCD3500 Shutter": Value Change {
            n279 = event-data() -> ("NewVal"=w289:bool)  [unwired: 1 in, 4 out]
            n280 = local read "CCD3500V Status"() -> (w290:bool)
            n281 = case shown="True" w290 {
              tunnel: w289 -> [_ w291]
              frame False {
              }
              frame True {
                n282 = stacked-sequence {
                  tunnel: w291 -> [w293]
                  frame #0 {
                    n283 = local read "CCD3500V Connection"() -> (w294:T2)
                    n284 = call "CCD Shutter.vi"("Shutter"=w293, "Comm Params"=w294) -> ("Error"=w292:bool)
                    n285 = local write "CCD3500 Shutter"(w292) -> ()
                  }
                }
              }
            }
          }
          event "Drive GoTo": Value Change {
            n286 = event-data() -> ("NewVal"=w295:bool)  [unwired: 1 in, 4 out]
            n287 = stacked-sequence {
              tunnel: w295 -> [_ w297 _]
              frame #0 {
                n288 = property on="Drive Running" class="Bool (strict)"("Blinking"=TRUE ("Blinkend")) -> ()  [unwired: 2 in, 2 out]
              }
              frame #1 {
                n289 = local read "Drive Status"() -> (w299:bool)
                n290 = And(x=w299, y=w297) -> (x .and. y?=w298:bool)
                n291 = case shown="True" w298 {
                  frame False {
                  }
                  frame True {
                    n292 = local read "Drive New Positions"() -> (w300:T11)
                    n293 = local read "Drive Connection"() -> (w301:T10)
                    n294 = control-ref of="Drive Running"() -> (w302:refnum<vi>)
                    n295 = call "ESA-C Move Absolute.vi"("Running"=w302, "Drive New Abs. Positions"=w300, "Drive Connection Settings"=w301) -> ()  [unwired: 2 in]
                  }
                }
              }
              frame #2 {
                w304 = FALSE ("Blinkend")
                n296 = local write "Drive GoTo"(w304) -> ()
                n297 = property on="Drive Running" class="Bool (strict)"("Blinking"=w304) -> ()  [unwired: 2 in, 2 out]
                n298 = property on="Read Drive" class="Bool (strict)"("Val(Sgnl)"=TRUE ("Wert (signalisierend)")) -> ()  [unwired: 2 in, 2 out]
              }
            }
          }
          event Value Change {
            n299 = event-data() -> ("NewVal"=w306:bool)  [unwired: 1 in, 4 out]
            n300 = local read "Drive Status"() -> (w307:bool)
            n301 = And(x=w307, y=w306) -> (x .and. y?=w305:bool)
            n302 = case shown="True" w305 {
              frame False {
              }
              frame True {
                n303 = stacked-sequence {
                  seq-local: [w308 _ _ _] -> [_ w324 _ _]
                  frame #0 {
                    # "Move and Read"
                    n304 = flat-sequence {
                      tunnel: [w315] -> w311
                      tunnel: [w312] -> w310
                      tunnel: w311 -> [w317]
                      tunnel: w310 -> [w318]
                      tunnel: [w316] -> w309
                      tunnel: w309 -> [w323]
                      tunnel: [w323] -> w308
                      frame #0 {
                        n305 = local read "Drive Live Controls"() -> (w312:T15)
                        n306 = local read "Drive Connection"() -> (w313:T10)
                        n307 = control-ref of="Drive Running"() -> (w314:refnum<vi>)
                        n308 = call "ESA-C Live Control.vi"("Running"=w314, "Drive Live Controls"=w312, "Drive Connection Settings"=w313) -> ("Reset Switches"=w315:bool)  [unwired: 1 in]
                      }
                      frame #1 {
                        n309 = case shown="True" w317 {
                          tunnel: w318 -> [w319 w322]
                          tunnel: [w319 w321] -> w316
                          frame False {
                          }
                          frame True {
                            w320 = FALSE ("Move Out")
                            n310 = Bundle By Name(cluster=w322, "Move Home"=w320, "Move Down"=w320, "Move Up"=w320, "Move Left"=w320, "Move Right"=w320, "Move Out"=w320, "Move In"=w320) -> (w321:T15)
                          }
                        }
                      }
                      frame #2 {
                        n311 = local write "Drive Live Controls"(w323) -> ()
                      }
                    }
                  }
                  frame #1 {
                    # "Snapshot"
                    n312 = Unbundle By Name(w324) -> ("Snapshot"=w327:bool)
                    n313 = case shown="True" w327 {
                      selector: w327 -> [w328 _]
                      tunnel: [w328 FALSE] -> w326
                      frame False {
                      }
                      frame True {
                        n314 = call "Video Snapshot.vi"() -> ()  [unwired: 11 in, 1 out]
                      }
                    }
                    n315 = Bundle By Name(cluster=w324, "Snapshot"=w326) -> (w325:T15)
                    n316 = local write "Drive Live Controls"(w325) -> ()
                  }
                  frame #2 {
                    n317 = local write "Copy Drive Target"(TRUE ("Copy Drive Target")) -> ()
                  }
                  frame #3 {
                    n318 = property on="Read Drive" class="Bool (strict)"("Val(Sgnl)"=TRUE ("Wert (signalisierend)")) -> ()  [unwired: 2 in, 2 out]
                  }
                }
              }
            }
          }
          event "Spectrum Save": Value Change {
            n319 = event-data() -> ("NewVal"=w332:bool)  [unwired: 1 in, 4 out]
            n320 = stacked-sequence {
              tunnel: w332 -> [w333 _]
              frame #0 {
                n321 = case shown="True" w333 {
                  frame False {
                  }
                  frame True {
                    n322 = local read "Spectrum"() -> (w337:cluster{dbl[], dbl[]}[])
                    n323 = local read "CCD3500 Temperature"() -> (w341:dbl)
                    n324 = local read "ITC503 Current Values"() -> (w342:T7)
                    n325 = local read "Drive Current Values"() -> (w343:T9)
                    n326 = local read "iHR Current Values"() -> (w345:T14)
                    n327 = local read "Spectra Settings"() -> (w344:T12)
                    n328 = Index Array(array=w337, index=0 ("Index")) -> (element=w335:cluster{dbl[], dbl[]})
                    n329 = Unbundle(w335) -> (w348:dbl[], w347:dbl[])
                    n330 = Build Array(w348, w347) -> (w346:dbl[][])
                    n331 = call "Export_spectrumFileName.vi"("ITC503 Current Values"=w342, "iHR Current Values"=w345, "Spectra Settings"=w344, "Drive Current Values"=w343, "CCD3500 Temperature"=w341) -> ("Filename"=w340:string)
                    n332 = local read "Spectrum Autosave"() -> (w338:bool)
                    n333 = local read "Auto Folder"() -> (w334:path)
                    n334 = call "Export_2DtoTxt v10.2.0.vi"("Auto Folder"=w334, "Auto?"=w338, "Data (2D)"=w346, "Export Type"="Spectrum", "Filename"=w340) -> ()  [unwired: 1 in]
                  }
                }
              }
              frame #1 {
                n335 = local write "Spectrum Save"(FALSE ("Spectrum Save")) -> ()
              }
            }
          }
          event "Spectrum Load": Value Change {
            n336 = event-data() -> ("NewVal"=w350:bool)  [unwired: 1 in, 4 out]
            n337 = stacked-sequence {
              tunnel: w350 -> [w351 _]
              frame #0 {
                n338 = case shown="True" w351 {
                  frame False {
                  }
                  frame True {
                    n339 = local read "Spectrum"() -> (w354:cluster{dbl[], dbl[]}[])
                    n340 = call "Load Spectrum.vi"() -> ("Graph Cluster"=w352:cluster{dbl[], dbl[]})  [unwired: 3 in, 2 out]
                    n341 = Build Array (concatenate)(w354, w352) -> (w353:cluster{dbl[], dbl[]}[])
                    n342 = local write "Spectrum"(w353) -> ()
                  }
                }
              }
              frame #1 {
                n343 = local write "Spectrum Load"(FALSE ("Spectrum Load")) -> ()
              }
            }
          }
          event "Spectrum Autosave": Value Change {
            n344 = event-data() -> ("NewVal"=w357:bool)  [unwired: 1 in, 4 out]
            n345 = case shown="True" w357 {
              tunnel: [path "" w363] -> w356
              frame False {
              }
              frame True {
                n346 = call "File Dialog"("prompt"="Choose Save Folder") -> ("selected path"=w365:path, "cancelled"=w359:bool, "error out"=w361:errorcluster)  [unwired: 11 in, 1 out]
                n347 = call <vilib>:"Simple Error Handler.vi"("error in (no error)"=w361) -> ("error?"=w360:bool)  [unwired: 4 in, 4 out]
                n348 = Or(x=w359, y=w360) -> (x .or. y?=w362:bool)
                n349 = case shown="True" w362 {
                  tunnel: w365 -> [w366 _]
                  tunnel: [w366 path ""] -> w363
                  frame False {
                  }
                  frame True {
                    n350 = local write "Spectrum Autosave"(FALSE ("Spectrum Autosave")) -> ()
                  }
                }
              }
            }
            n351 = local write "Auto Folder"(w356) -> ()
          }
          event "Spectrum Maximize": Value Change {
            n352 = event-data() -> ("NewVal"=w369:bool)  [unwired: 1 in, 4 out]
            n353 = case shown="True" w369 {
              frame False {
                n354 = local read "Spectrum Properties"() -> (w372:cluster{"Position":T1, "Plot Area Size":T1})
                n355 = Unbundle(w372) -> ("Position"=w371:T1, "Plot Area Size"=w370:T1)
                n356 = stacked-sequence {
                  tunnel: w371 -> [_ w374]
                  tunnel: w370 -> [w373 _]
                  frame #0 {
                    n357 = property on="Spectrum" class="XYGraph (strict)"("Plot Area Size"=w373) -> ()  [unwired: 2 in, 2 out]
                  }
                  frame #1 {
                    n358 = property on="Spectrum" class="XYGraph (strict)"("Position"=w374) -> ()  [unwired: 2 in, 2 out]
                  }
                }
              }
              frame True {
                n359 = property on="Spectrum" class="XYGraph (strict)"() -> ("Bounds"=w395:T1, "Plot Area Size"=w394:T1, "Position"=w392:T23)  [unwired: 2 in, 2 out]
                n360 = Bundle("Position"=w392, "Plot Area Size"=w394) -> (w393:cluster{"Position":T23, "Plot Area Size":T1})  [unwired: 1 in]
                n361 = Unbundle By Name(w395) -> ("Width"=w399:u32, "Height"=w400:u32)
                n362 = Unbundle By Name(w394) -> ("Width"=w402:u32, "Height"=w401:u32)
                n363 = property on="Register" class="TabCtl (strict)"() -> ("Bounds"=w398:T1, "Position"=w387:T23, "Width"=w378:u32, "Height"=w377:u32)  [unwired: 2 in, 2 out]
                n364 = local write "Spectrum Properties"(w393) -> ()
                n365 = Subtract(x=w399, y=w402) -> (x-y=w391:u32)
                n366 = Subtract(x=w400, y=w401) -> (x-y=w388:u32)
                n367 = Add(x=w391, y=u32 25) -> (x+y=w390:u32)
                n368 = Add(x=w388, y=u32 70) -> (x+y=w389:u32)
                n369 = Subtract(x=w378, y=w390) -> (x-y=w397:u32)
                n370 = Subtract(x=w377, y=w389) -> (x-y=w396:u32)
                n371 = Bundle By Name(cluster=w398, "Width"=w397, "Height"=w396) -> (w375:T1)
                n372 = Unbundle By Name(w387) -> ("Left"=w386:i32, "Top"=w383:i32)
                n373 = Add(x=w386, y=20) -> (x+y=w385:i32)
                n374 = Add(x=w383, y=50) -> (x+y=w384:i32)
                n375 = Bundle By Name(cluster=w387, "Left"=w385, "Top"=w384) -> (w376:T23)
                n376 = stacked-sequence {
                  tunnel: w376 -> [w403 _]
                  tunnel: w375 -> [_ w404]
                  frame #0 {
                    n377 = property on="Spectrum" class="XYGraph (strict)"("Position"=w403) -> ()  [unwired: 2 in, 2 out]
                  }
                  frame #1 {
                    n378 = property on="Spectrum" class="XYGraph (strict)"("Plot Area Size"=w404) -> ()  [unwired: 2 in, 2 out]
                  }
                }
              }
            }
          }
          event "Mapping Start": Value Change {
            n379 = event-data() -> ("NewVal"=w405:bool)  [unwired: 1 in, 4 out]
            n380 = case shown="True" w405 {
              frame False {
              }
              frame True {
                n381 = stacked-sequence {
                  frame #0 {
                    n382 = property on="Measurement Running" class="Bool (strict)"("Blinking"=TRUE ("Blinkend")) -> ()  [unwired: 2 in, 2 out]
                  }
                  frame #1 {
                    w421 = FALSE ("Simulate Drive")
                    n383 = local read "CCD3500V Connection"() -> (w417:T2)
                    n384 = local read "CCD3500 Temperature"() -> (w419:dbl)
                    n385 = local read "ITC503 Current Values"() -> (w414:T7)
                    n386 = local read "Drive Current Values"() -> (w412:T9)
                    n387 = local read "iHR Current Values"() -> (w413:T14)
                    n388 = local read "Wavelengths (nm)"() -> (w415:dbl[])
                    n389 = local read "Drive Connection"() -> (w416:T10)
                    n390 = local read "CCD3500V Status"() -> (w408:bool)
                    n391 = local read "Spectra Settings"() -> (w418:T12)
                    n392 = local read "Drive Status"() -> (w410:bool)
                    n393 = Not(x=w410) -> (.not. x?=w409:bool)
                    n394 = Not(x=w408) -> (.not. x?=w407:bool)
                    n395 = Bundle By Name(cluster=T20 {"CCD3000 Connection"={"Comm Interface"=1, "BUS"=0, "Address"=5, "Com Port"=1}, "Drive Connection Settings"={"Objective GPIB-Port"=4, "Stage GPIB-Port"=4, "Drive Selector"=0, "Drive Velocity (V/s)"=5.0}, "ITC503 Current Values"={"ITC503 Heater"=0.0, "ITC503 Temperature"=0.0, "ITC503 P"=0.0, "ITC503 I"=0.0, "ITC503 D"=0.0, "ITC503 Setpoint"=0.0, "ITC503 Gradient"=0.0, "ITC503 Heater Auto"=FALSE, "ITC503 PID Auto"=FALSE}, "Wavelengths (nm)"=[], "Drive Current Values"={"Voltages"={"Drive X Voltage"=0.0, "Drive Y Voltage"=0.0, "Drive Z Voltage"=0.0}, "Position"={"Drive X Position"=0.0, "Drive Y Position"=0.0, "Drive Z Position"=0.0}}, "iHR Current Values"={"iHR 550 Front Entrance"=0.0, "iHR550 Side Exit"=0.0, "iHR550 Wavelength"=897.9988, "iHR550 Exit Mirror"=2, "iHR550 Grating"="1", "Grating Index"=1}, "Spectra Settings"={"Integration Time"=1.0, "Repetitions"=1, "Mapping Spectra"=TRUE}, "CCD3500 Temperature"=0.0, "Simulate Drive 2"=FALSE, "Simulate Spectra 2"=FALSE} ("Input Parameters"), "CCD3000 Connection"=w417, "Drive Connection Settings"=w416, "ITC503 Current Values"=w414, "Wavelengths (nm)"=w415, "Drive Current Values"=w412, "iHR Current Values"=w413, "Spectra Settings"=w418, "CCD3500 Temperature"=w419, "Simulate Drive 2"=w409, "Simulate Spectra 2"=w407) -> (w420:T20)
                    n396 = call "Mapping v10.2.2.vi"("Simulate Spectra"=w421, "Simulate Drive"=w421, "Input Parameters"=w420) -> ()  [unwired: 9 in]
                  }
                  frame #2 {
                    # "reinitialize CCD after mapping"
                    n397 = local read "CCD3500V Connection"() -> (w422:T2)
                    n398 = local read "Spectra Settings"() -> (w424:T12)
                    n399 = call "CCD3000 Prepare Acquisition.vi"("Mapping Spectra Settings"=w424, "Comm Params"=w422) -> ()  [unwired: 4 in]
                    n400 = Unbundle By Name(w424) -> ("Integration Time"=w423:dbl)
                    n401 = local write "Int. Time Temp"(w423) -> ()
                  }
                  frame #3 {
                    # "reinitialize Drive after mapping"
                    n402 = stacked-sequence {
                      frame #0 {
                        # "read current values"
                        n403 = property on="Read Drive" class="Bool (strict)"("Val(Sgnl)"=TRUE ("Value (Signaling)")) -> ()  [unwired: 2 in, 2 out]
                      }
                      frame #1 {
                        # "mirror to \"GoTo\" fields"
                        n404 = local write "Copy Drive Target"(TRUE ("Copy Drive Target")) -> ()
                      }
                    }
                  }
                  frame #4 {
                    w427 = FALSE ("Mapping Start")
                    n405 = local write "Mapping Start"(w427) -> ()
                    n406 = property on="Measurement Running" class="Bool (strict)"("Blinking"=w427) -> ()  [unwired: 2 in, 2 out]
                  }
                }
              }
            }
          }
        }
      }
    }
    frame #3 {
      # "Close Connections"
      n407 = control-ref of="Dieses VI"() -> (w428:refnum<vi>)
      n408 = invoke class="VI" method="Default Vals.Reinit All"(reference=w428) -> ()  [unwired: 2 in, 3 out]
    }
  }
